vi "HXG2_SAVE-PID_gains.vi"(8 "error in":errorcluster, 11 "PID Gains In":T1) -> (0 "error out":errorcluster)   [LabVIEW 2012]
uses:
  <vilib>/Utility/file.llb/Write To Spreadsheet File (DBL).vi
  Controls/HXG2_PIDgains_Array.ctl
panel:
  out "size(s)":i32
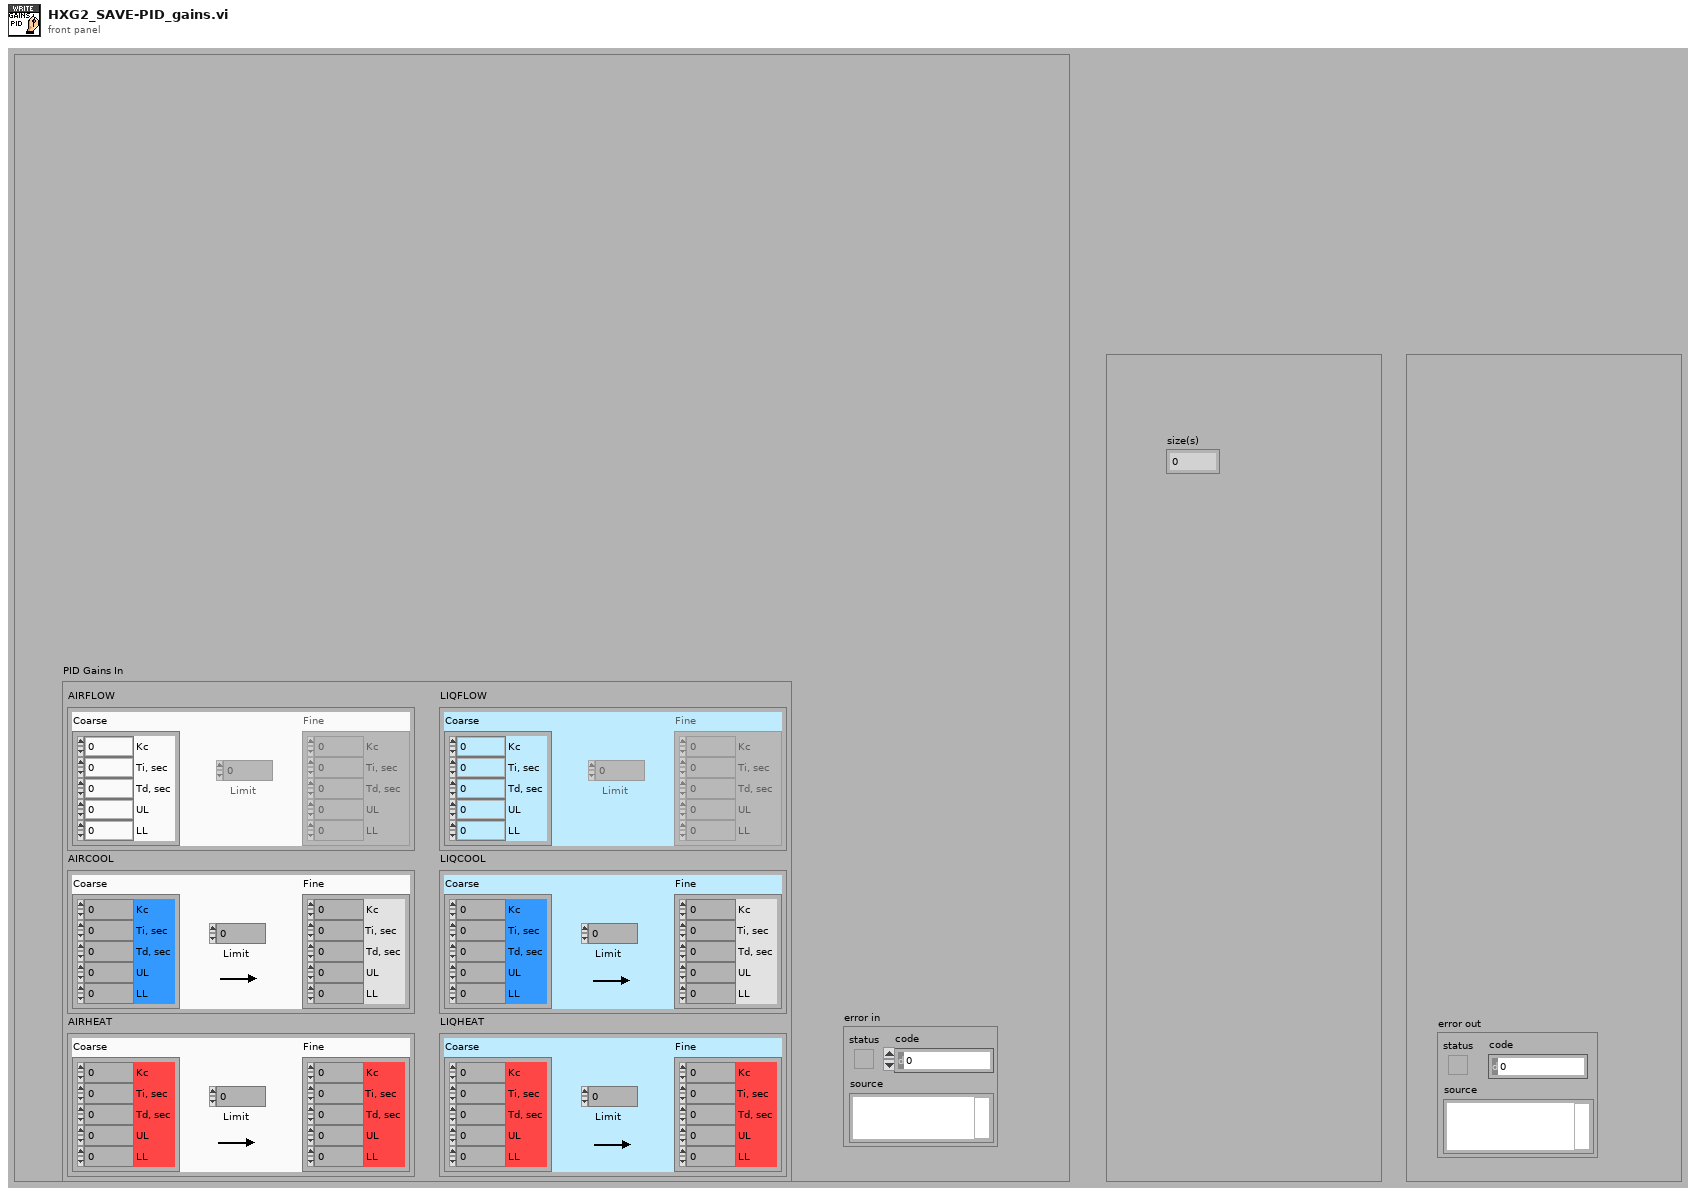
[diagram p1: front panel]
types:
  T1 = typedef "HXG2_PIDgains_Array.ctl" = cluster{"AIRFLOW":cluster{"Coarse":cluster{"Kc":dbl, "Ti, sec":dbl, "Td, sec":dbl, "UL":dbl, "LL":dbl}, "Fine":cluster{"Kc":dbl, "Ti, sec":dbl, "Td, sec":dbl, "UL":dbl, "LL":dbl}, "Limit":dbl}, "AIRCOOL":cluster{"Coarse":cluster{"Kc":dbl, "Ti, sec":dbl, "Td, sec":dbl, "UL":dbl, "LL":dbl}, "Fine":cluster{"Kc":dbl, "Ti, sec":dbl, "Td, sec":dbl, "UL":dbl, "LL":dbl}, "Limit":dbl}, "AIRHEAT":cluster{"Coarse":cluster{"Kc":dbl, "Ti, sec":dbl, "Td, sec":dbl, "UL":dbl, "LL":dbl}, "Fine":cluster{"Kc":dbl, "Ti, sec":dbl, "Td, sec":dbl, "UL":dbl, "LL":dbl}, "Limit":dbl}, "LIQFLOW":cluster{"Coarse":cluster{"Kc":dbl, "Ti, sec":dbl, "Td, sec":dbl, "UL":dbl, "LL":dbl}, "Fine":cluster{"Kc":dbl, "Ti, sec":dbl, "Td, sec":dbl, "UL":dbl, "LL":dbl}, "Limit":dbl}, "LIQCOOL":cluster{"Coarse":cluster{"Kc":dbl, "Ti, sec":dbl, "Td, sec":dbl, "UL":dbl, "LL":dbl}, "Fine":cluster{"Kc":dbl, "Ti, sec":dbl, "Td, sec":dbl, "UL":dbl, "LL":dbl}, "Limit":dbl}, "LIQHEAT":cluster{"Coarse":cluster{"Kc":dbl, "Ti, sec":dbl, "Td, sec":dbl, "UL":dbl, "LL":dbl}, "Fine":cluster{"Kc":dbl, "Ti, sec":dbl, "Td, sec":dbl, "UL":dbl, "LL":dbl}, "Limit":dbl}}
  T2 = cluster{"Kc":dbl, "Ti, sec":dbl, "Td, sec":dbl, "UL":dbl, "LL":dbl}
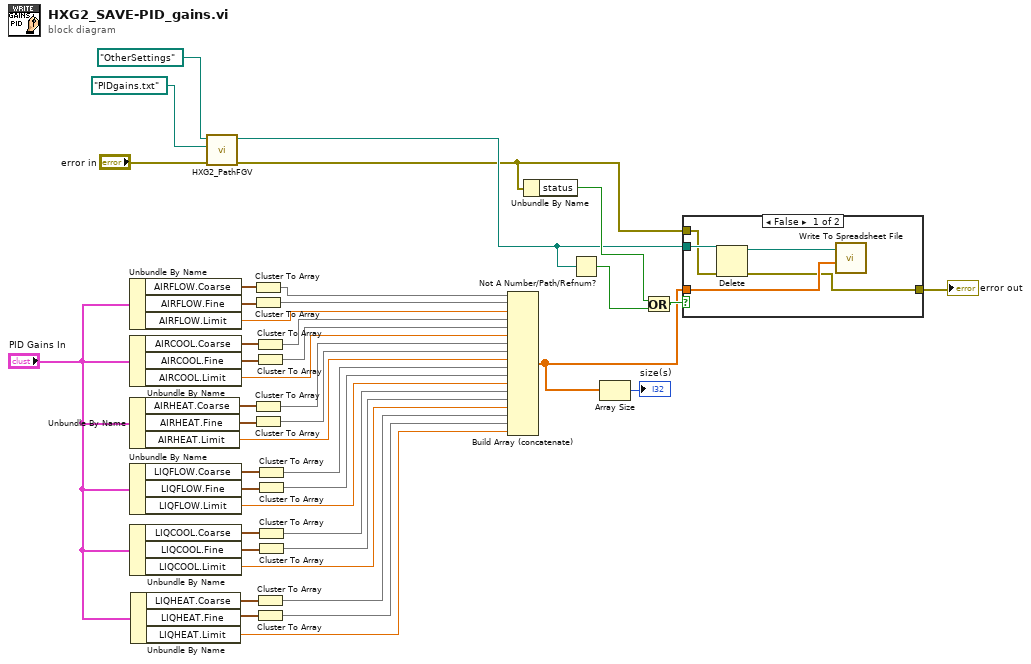
[diagram p0: block diagram]
diagram:
  n1 = Unbundle By Name("PID Gains In") -> ("AIRFLOW.Coarse"=w38:T2, "AIRFLOW.Fine"=w36:T2, "AIRFLOW.Limit"=w34:dbl)
  n2 = Unbundle By Name("PID Gains In") -> ("AIRCOOL.Coarse"=w33:T2, "AIRCOOL.Fine"=w32:T2, "AIRCOOL.Limit"=w29:dbl)
  n3 = Unbundle By Name("PID Gains In") -> ("AIRHEAT.Coarse"=w27:T2, "AIRHEAT.Fine"=w28:T2, "AIRHEAT.Limit"=w24:dbl)
  n4 = Unbundle By Name("PID Gains In") -> ("LIQFLOW.Coarse"=w23:T2, "LIQFLOW.Fine"=w22:T2, "LIQFLOW.Limit"=w19:dbl)
  n5 = Unbundle By Name("PID Gains In") -> ("LIQCOOL.Coarse"=w17:T2, "LIQCOOL.Fine"=w18:T2, "LIQCOOL.Limit"=w14:dbl)
  n6 = Unbundle By Name("PID Gains In") -> ("LIQHEAT.Coarse"=w13:T2, "LIQHEAT.Fine"=w12:T2, "LIQHEAT.Limit"=w9:dbl)
  n7 = call "HXG2_PathFGV.vi"("error in (no error)"="error in", "File Name"=path "PIDgains.txt", "Folder Name"=path "OtherSettings") -> ("error out"=w1:errorcluster, "File path"=w3:path)  [unwired: 5 in, 2 out]
  n8 = Cluster To Array(cluster=w38) -> (array=w37:dbl[])
  n9 = Cluster To Array(cluster=w36) -> (array=w35:dbl[])
  n10 = Cluster To Array(cluster=w27) -> (array=w26:dbl[])
  n11 = Cluster To Array(cluster=w28) -> (array=w25:dbl[])
  n12 = Cluster To Array(cluster=w33) -> (array=w31:dbl[])
  n13 = Cluster To Array(cluster=w32) -> (array=w30:dbl[])
  n14 = Cluster To Array(cluster=w13) -> (array=w11:dbl[])
  n15 = Cluster To Array(cluster=w12) -> (array=w10:dbl[])
  n16 = Cluster To Array(cluster=w23) -> (array=w21:dbl[])
  n17 = Cluster To Array(cluster=w22) -> (array=w20:dbl[])
  n18 = Cluster To Array(cluster=w17) -> (array=w16:dbl[])
  n19 = Cluster To Array(cluster=w18) -> (array=w15:dbl[])
  n20 = Build Array (concatenate)(w37, w35, w34, w31, w30, w29, w26, w25, w24, w21, w20, w19, w16, w15, w14, w11, w10, w9) -> (w40:dbl[])
  n21 = Unbundle By Name(w1) -> ("status"=w6:bool)
  n22 = Not A Number/Path/Refnum?(number/path/refnum=w3) -> (NaN/Path/Refnum?=w7:bool)
  n23 = Array Size(array=w40) -> (size(s)=→"size(s)":i32)
  n24 = Or(x=w6, y=w7) -> (x .or. y?=w42:bool)
  n25 = case shown="False" w42 {
    tunnel: w40 -> [w47 _]
    tunnel: w3 -> [w46 _]
    tunnel: w1 -> [w44 w48]
    tunnel: [w43 w48] -> w41
    frame False {
      n26 = Delete(path (use dialog)=w46, error in=w44) -> (deleted path=w45:path, error out=w43:errorcluster)  [unwired: 4 out]
      n27 = call-poly <vilib>:"Write To Spreadsheet File.vi"("1D data"=w47, "file path (dialog if empty)"=w45) -> ()  [unwired: 4 in, 3 out]
    }
    frame True {
    }
  }
  "error out" <- w41
